vi "Initialize.vi"(6 "Loader":refnum<class "Loader.lvclass">, 7 "Data":refnum<class "Datum.lvclass">, 8 "Error In":errorcluster, 10 "Writer":refnum<class "Writer.lvclass">, 11 "Renderer In":refnum<class "Renderer.lvclass">) -> (0 "Error Out":errorcluster, 3 "Renderer Out":refnum<class "Renderer.lvclass">)   [LabVIEW 2018, in "Toolkit.lvlib" / "Renderer.lvclass"]
uses:
  Renderer.lvclass
  Data/Datum/Datum.lvclass
  Loaders/Loader/Loader.lvclass
  Writers/Writer/Writer.lvclass
  Renderer.lvclass/Renderer.ctl
  Loaders/File/File.lvclass
  D:/Users/cfield/Code/Field R&D Services/Labstache/src/Toolkit/Low-Level/Loaders/Loader/Loader.lvclass
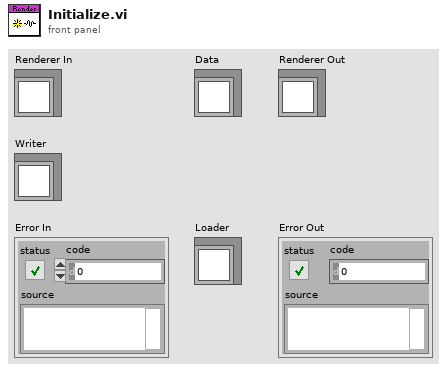
[diagram p1: front panel]
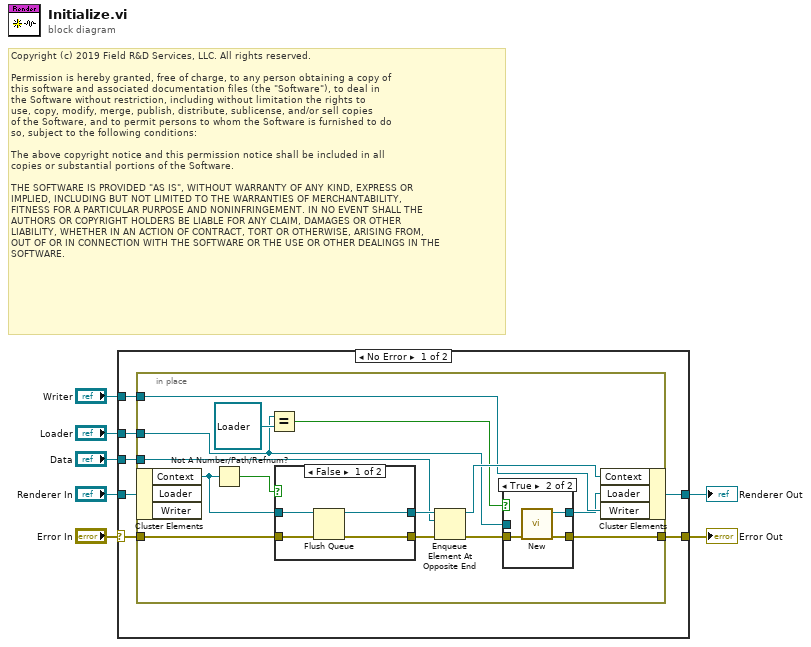
[diagram p0: block diagram]
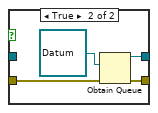
[diagram p3: hidden frame]
diagram:
  # "Copyright (c) 2019 Field R&D Services, LLC. All rights reserved.\n\nPermission is hereby granted, free of charge, to any person obtaining a copy of\nthis software and associated documentation files (the \"Software\"), to deal in\nthe Software without restriction, including without limitation the rights to\nuse, copy, modify, merge, publish, distribute, sublicense, and/or sell copies\nof the Software, and to permit persons to whom the Software is furnished to do\nso, subject to the following conditions:\n\nThe above copyright notice and this permission notice shall be included in all\ncopies or substantial portions of the Software.\n\nTHE SOFTWARE IS PROVIDED \"AS IS\", WITHOUT WARRANTY OF ANY KIND, EXPRESS OR\nIMPLIED, INCLUDING BUT NOT LIMITED TO THE WARRANTIES OF MERCHANTABILITY,\nFITNESS FOR A PARTICULAR PURPOSE AND NONINFRINGEMENT. IN NO EVENT SHALL THE\nAUTHORS OR COPYRIGHT HOLDERS BE LIABLE FOR ANY CLAIM, DAMAGES OR OTHER\nLIABILITY, WHETHER IN AN ACTION OF CONTRACT, TORT OR OTHERWISE, ARISING FROM,\nOUT OF OR IN CONNECTION WITH THE SOFTWARE OR THE USE OR OTHER DEALINGS IN THE\nSOFTWARE."
  n1 = case shown="No Error" "Error In" {
    selector: "Error In" -> [w13 w43]
    tunnel: [w14 w43] -> w7
    tunnel: "Renderer In" -> [w12 w42]
    tunnel: [w11 w42] -> w3
    tunnel: "Data" -> [w10 _]
    tunnel: "Loader" -> [w9 _]
    tunnel: "Writer" -> [w8 _]
    frame No Error {
      n2 = in-place {
        in-place-border: [w17] -> w14
        in-place-border: w13 -> [w28]
        in-place-border: w10 -> [w22]
        in-place-border: w9 -> [w15]
        in-place-border: w8 -> [w21]
        n3 = in-place-cluster #1(w12) -> ("Context"=w26:refnum<queue>)  [unwired: 2 out]
        n4 = Not A Number/Path/Refnum?(number/path/refnum=w26) -> (NaN/Path/Refnum?=w27:bool)
        n5 = Equal?(x=w15, y=refnum<class "Loader.lvclass"> refnum ("Loader")) -> (x = y?=w19:bool)
        n6 = case shown="False" w27 {
          tunnel: [w34 w40] -> w23
          tunnel: w28 -> [w35 w39]
          tunnel: [w36 w38] -> w25
          tunnel: w26 -> [w37 _]
          frame False {
            n7 = Flush Queue(queue=w37, error in (no error)=w35) -> (queue out=w36:refnum<queue>, error out=w34:errorcluster)  [unwired: 1 out]
          }
          frame True {
            n8 = Obtain Queue(element data type=refnum<class "Datum.lvclass"> refnum ("Toolkit.lvlib:Data.lvlib:Abstract.lvclass"), error in (no error)=w39) -> (queue out=w38:refnum<queue>, error out=w40:errorcluster)  [unwired: 3 in, 1 out]
          }
        }
        n9 = Enqueue Element At Opposite End(queue=w25, element=w22, error in (no error)=w23) -> (queue out=w24:refnum<queue>, error out=w18:errorcluster)  [unwired: 1 in, 1 out]
        n10 = case shown="True" w19 {
          tunnel: [w30 w33] -> w16
          tunnel: w18 -> [w29 w32]
          tunnel: w15 -> [w30 _]
          tunnel: [w29 w31] -> w17
          frame False {
          }
          frame True {
            n11 = call "New.vi"("Error In"=w32) -> ("Error Out"=w31:errorcluster, "File"=w33:refnum<class "File.lvclass">)  [unwired: 9 in]
          }
        }
        n12 = in-place-cluster #1("Context"=w24, "Loader"=w16, "Writer"=w21) -> (w11:refnum<class "Renderer.lvclass">)
      }
    }
    frame Error {
    }
  }
  "Error Out" <- w7
  "Renderer Out" <- w3
